vi "New User.vi"(8 "Error in":errorcluster) -> (0 "Error out":errorcluster)   [LabVIEW 2019, in "User Lib.lvlib"]
uses:
  User Lib.lvlib
  <vilib>/addons/database/Connection.llb/DB Tools Open Connec (String).vi
  <vilib>/addons/database/_DB Variant To Data/Database Variant To Data.xnode
  <vilib>/addons/database/NI_Database_API.lvlib
  database.lvlib
panel:
  in  "Cancel":bool
  in  "OK":bool
  in  "Is Admin?":enum32{"Yes", "No"}(radio)
  in  "Full Name":string
  in  "Confirm Password":string
  in  "Password":string
  in  "Username":string
  # "New User"
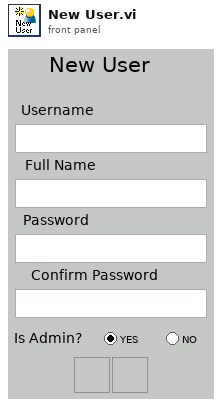
[diagram p1: front panel]
types:
  T1 = typedef "NI_Database_API.lvlib/Conn ObjectReference.ctl" = refnum<k1>
  T2 = cluster{"Username":string, "Full Name":string, "Password":string, string}
  T3 = cluster{i32, "date/time string":string, "date/time string":string, string}
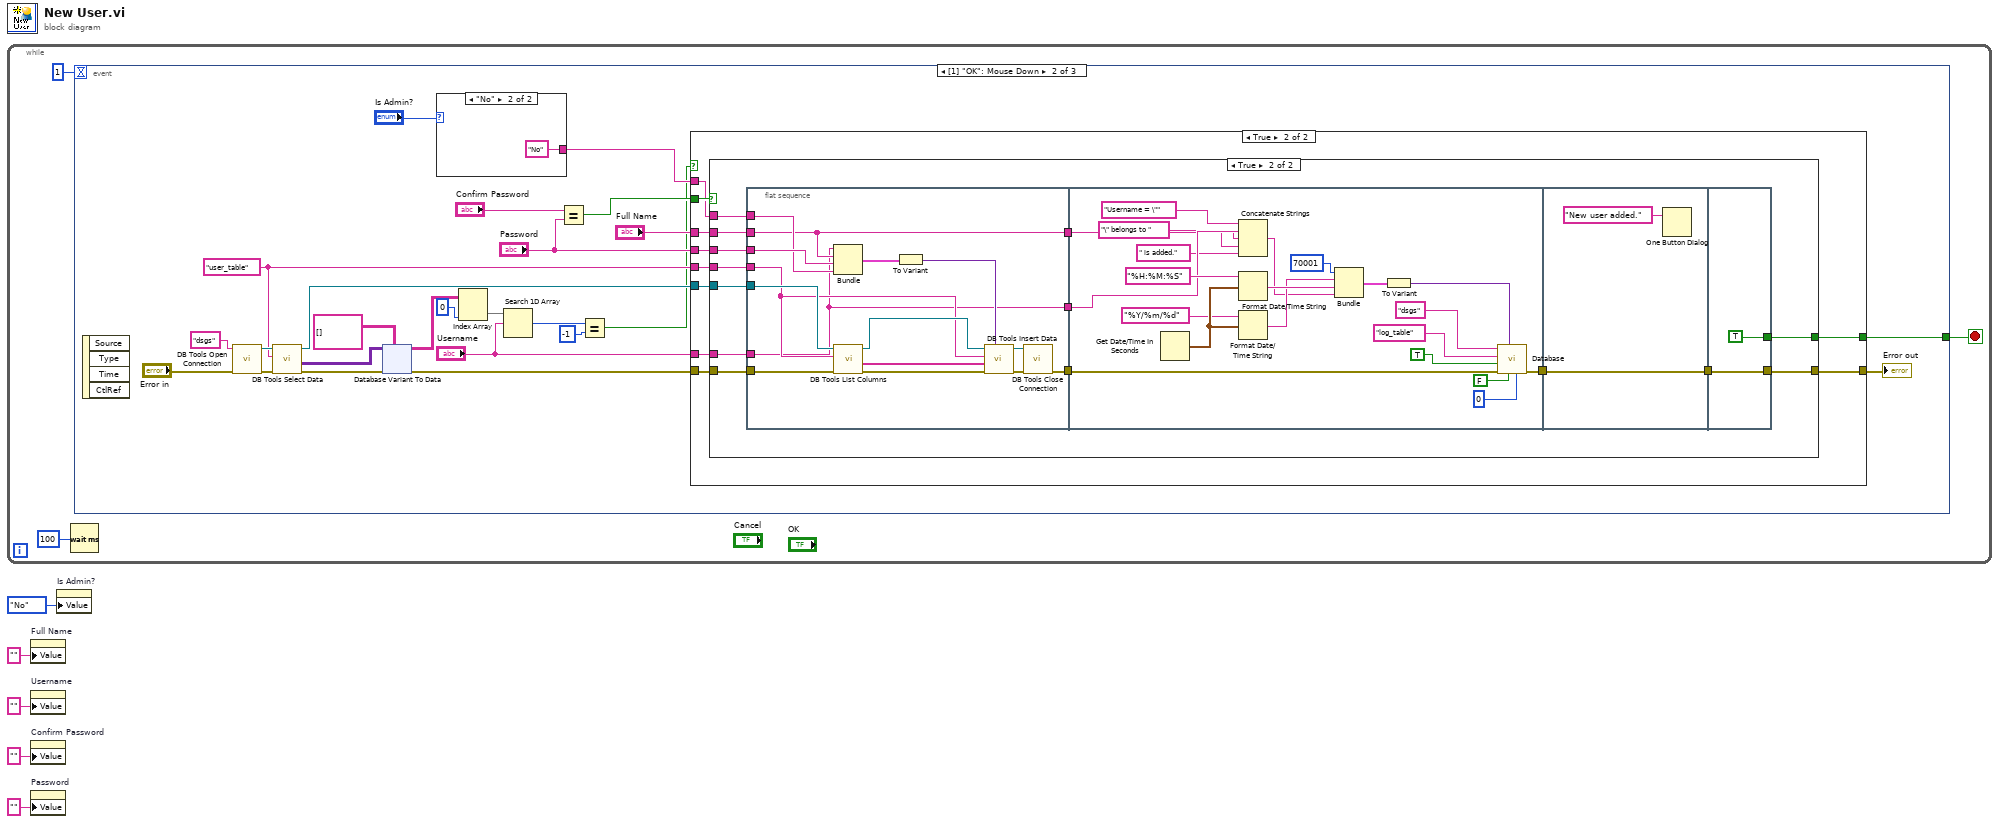
[diagram p0: block diagram]
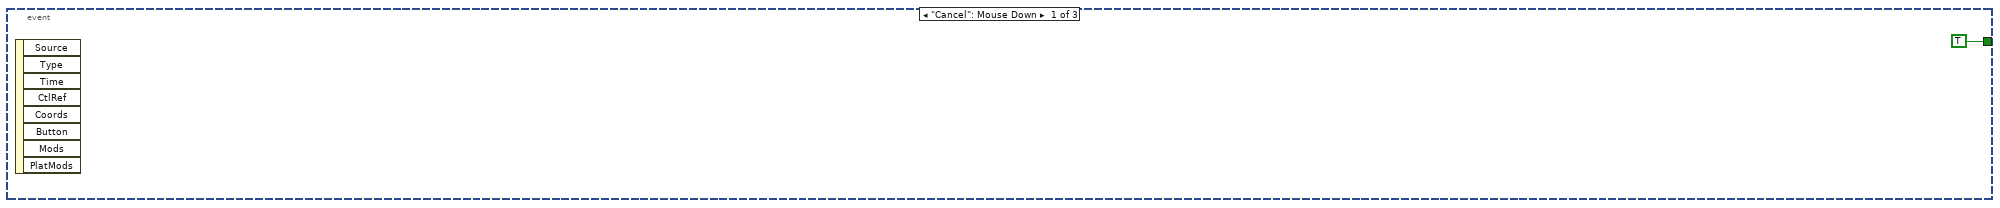
[diagram p2: hidden frame]
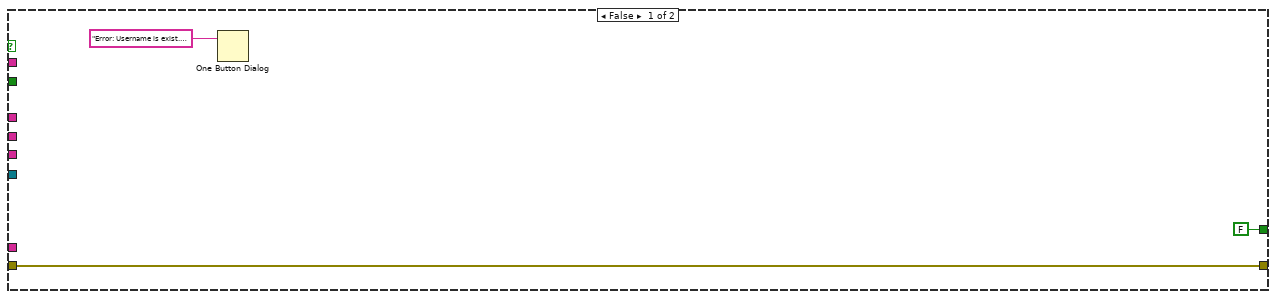
[diagram p3: hidden frame]
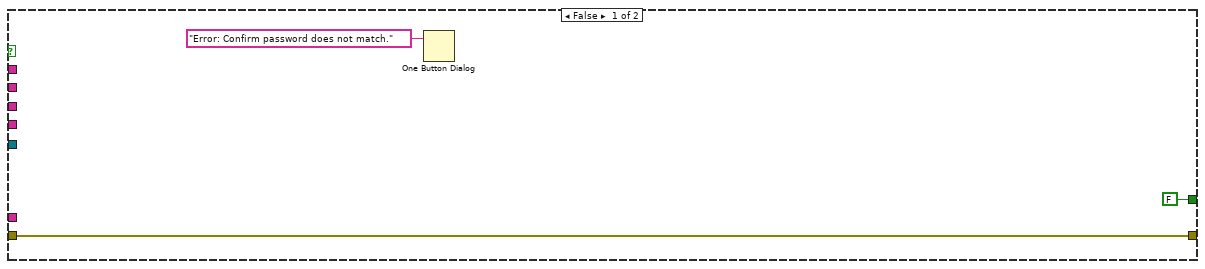
[diagram p4: hidden frame]
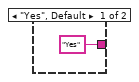
[diagram p5: hidden frame]
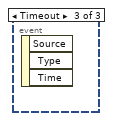
[diagram p6: hidden frame]
diagram:
  n1 = while {
    stop <- w7 stop-if-true
    n2 = Wait (ms)(milliseconds to wait=u32 100) -> ()  [unwired: 1 out]
    n3 = event shown="[1] \"OK\": Mouse Down" {
      selector: _ -> [_ _ _]
      dyn-events: _ -> [_ _ _]
      timeout: 1 -> [_ _ _]
      tunnel: [TRUE w28 _] -> w7
      event "Cancel": Mouse Down {
        n4 = event-data() -> ()  [unwired: 1 in, 8 out]
      }
      event "OK": Mouse Down {
        w22 = "user_table" ("Heat Table Name")
        n5 = event-data() -> ()  [unwired: 1 in, 4 out]
        n6 = call-poly <vilib>:"DB Tools Open Connection.vi"("error in (no error)"="Error in", "connection information"="dsgs" ("Connection Name")) -> ("error out"=w27:errorcluster, "connection reference"=w26:T1)  [unwired: 6 in]
        n7 = call <vilib>:"DB Tools Select Data.vi"("error in (no error)"=w27, "table"=w22, "connection reference"=w26) -> ("error out"=w20:errorcluster, "data"=w21:variant[][], "connection reference out"=w23:T1)  [unwired: 3 in]
        n8 = xnode "Database Variant To Data"("database variant"=w21, "error in (no error)"=w20, "type"=string[][] []) -> ("data"=w17:string[][], "error out"=w19:errorcluster)
        n9 = case shown="\"No\"" "Is Admin?" {
          tunnel: ["Yes" "No"] -> w29
          frame "Yes", Default {
          }
          frame "No" {
          }
        }
        n10 = Index Array(array=w17, index (col)=0 ("disabled index (col)")) -> (element=w15:string[])  [unwired: 1 in]
        n11 = Search 1D Array(1D array=w15, element="Username") -> (index of element=w13:i32)  [unwired: 1 in]
        n12 = Equal?(x="Confirm Password", y="Password") -> (x = y?=w32:bool)
        n13 = Equal?(x=w13, y=-1) -> (x = y?=w11:bool)
        n14 = case shown="True" w11 {
          tunnel: w32 -> [_ w47]
          tunnel: "Full Name" -> [_ w46]
          tunnel: "Password" -> [_ w45]
          tunnel: w29 -> [_ w44]
          tunnel: [FALSE w43] -> w28
          tunnel: w23 -> [_ w42]
          tunnel: [w36 w38] -> w10
          tunnel: w22 -> [_ w41]
          tunnel: w19 -> [w36 w40]
          tunnel: "Username" -> [_ w39]
          frame False {
            n15 = One Button Dialog(message="Error: Username is exist. Please choose another username.") -> ()  [unwired: 1 in, 1 out]
          }
          frame True {
            n16 = case shown="True" w47 {
              tunnel: w39 -> [_ w64]
              tunnel: w46 -> [_ w63]
              tunnel: w45 -> [_ w62]
              tunnel: w44 -> [_ w61]
              tunnel: [FALSE w57] -> w43
              tunnel: w40 -> [w48 w60]
              tunnel: w42 -> [_ w59]
              tunnel: [w48 w53] -> w38
              tunnel: w41 -> [_ w58]
              frame False {
                n17 = One Button Dialog(message="Error: Confirm password does not match.") -> ()  [unwired: 1 in, 1 out]
              }
              frame True {
                n18 = flat-sequence {
                  tunnel: w64 -> [w68]
                  tunnel: w63 -> [w69]
                  tunnel: w62 -> [w79]
                  tunnel: w61 -> [w78]
                  tunnel: w60 -> [w73]
                  tunnel: w59 -> [w72]
                  tunnel: w58 -> [w70]
                  tunnel: [w69] -> w56
                  tunnel: [w68] -> w55
                  tunnel: [w66] -> w54
                  tunnel: w56 -> [w85]
                  tunnel: w55 -> [w87]
                  tunnel: w54 -> [w82]
                  tunnel: [w81] -> w51
                  tunnel: [w101] -> w52
                  tunnel: w51 -> [w101]
                  tunnel: [TRUE] -> w57
                  tunnel: [w103] -> w53
                  tunnel: w52 -> [w103]
                  frame #0 {
                    n19 = Bundle("Username"=w68, "Full Name"=w69, "Password"=w79, w78) -> (w74:T2)  [unwired: 1 in]
                    n20 = call <vilib>:"DB Tools List Columns.vi"("error in (no error)"=w73, "table"=w70, "connection reference"=w72) -> ("error out"=w76:errorcluster, "columns"=w65:string[], "connection reference out"=w75:T1)  [unwired: 1 in, 1 out]
                    n21 = To Variant(anything=w74) -> (Variant=w77:variant)
                    n22 = call <vilib>:"DB Tools Insert Data.vi"("data"=w77, "error in (no error)"=w76, "columns"=w65, "table"=w70, "connection reference"=w75) -> ("error out"=w67:errorcluster, "connection reference out"=w71:T1)  [unwired: 5 in]
                    n23 = call <vilib>:"DB Tools Close Connection.vi"("error in (no error)"=w67, "connection reference"=w71) -> ("error out"=w66:errorcluster)  [unwired: 5 in]
                  }
                  frame #1 {
                    n24 = Get Date/Time In Seconds() -> (seconds since 1Jan1904=w96:timestamp)
                    n25 = Concatenate Strings("Username = \"" ("string"), w87, "\" belongs to " ("string"), w85, " is added." ("string")) -> (w83:string)
                    n26 = Format Date/Time String(time format string (%c)="%H:%M:%S", seconds (now)=w96) -> (date/time string=w98:string)  [unwired: 1 in]
                    n27 = Format Date/Time String(time format string (%c)="%Y/%m/%d", seconds (now)=w96) -> (date/time string=w97:string)  [unwired: 1 in]
                    n28 = Bundle(70001, "date/time string"=w97, "date/time string"=w98, w83) -> (w99:T3)  [unwired: 1 in]
                    n29 = To Variant(anything=w99) -> (Variant=w100:variant)
                    n30 = call "Database.vi"("Maximum Row"=u64 0 ("Storage Time (Day)"), "Delete row?"=FALSE, "Data"=w100, "Error in"=w82, "Auto Increment ID?"=TRUE, "Table"="log_table" ("table"), "Connection"="dsgs" ("table")) -> ("Error out"=w81:errorcluster)  [unwired: 4 in]
                  }
                  frame #2 {
                    n31 = One Button Dialog(message="New user added.") -> ()  [unwired: 1 in, 1 out]
                  }
                  frame #3 {
                  }
                }
              }
            }
          }
        }
        "Error out" <- w10
      }
      event Timeout {
        n32 = event-data() -> ()  [unwired: 1 in, 3 out]
      }
    }
  }
  n33 = property on="Full Name" class="Str"("Value"="" ("Full Name")) -> ()  [unwired: 2 in, 2 out]
  n34 = property on="Username" class="Str"("Value"="" ("Username")) -> ()  [unwired: 2 in, 2 out]
  n35 = property on="Confirm Password" class="Str"("Value"="" ("Username")) -> ()  [unwired: 2 in, 2 out]
  n36 = property on="Password" class="Str"("Value"="" ("Username")) -> ()  [unwired: 2 in, 2 out]
  n37 = property on="Is Admin?" class="RadioBtnsControl (strict)"("Value"=enum32{"Yes", "No"}."No" ("Is Admin?")) -> ()  [unwired: 2 in, 2 out]
